vi "GetOpenLastSavedFileWhenStarting.vi"(5 "error in (no error)":errorcluster) -> (15 "OpenLastSavedFileWhenStarting":bool, 19 "error out":errorcluster)   [LabVIEW 2012, in "UmlEditor.lvclass"]
uses:
  <resource>/Framework/Providers/Open_GDS/UML/UmlEditor_class/UmlEditor.lvclass
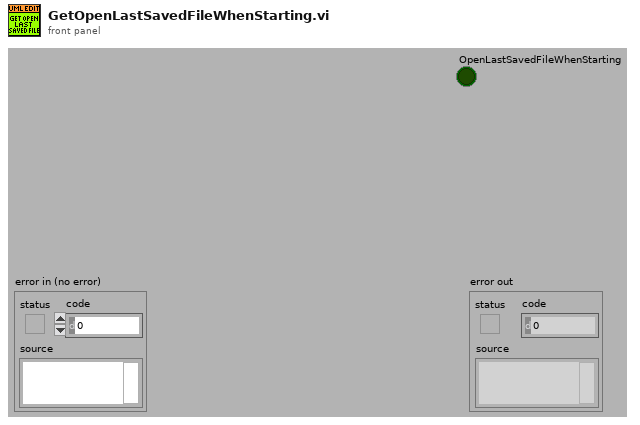
[diagram p1: front panel]
types:
  T1 = typedef "UmlEditor.lvclass/ObjectAttributes.ctl" = cluster{"ListeningQueueIn":refnum<queue>, "Event":refnum<user-event>, "UseProjectFolderAsBasePath":bool, "TypeSyncOption":bool, "Attr":string[], "ToolTip":cluster{"ToolTipOpen":bool, "LastToolTip":i32}, "ClassesToIgnore":string[], "UndoSize":i32, "OpenLastSavedFileWhenStarting":bool, "SyncOption":T2, "SyncTime(s)":i32, "Params":cluster{"IniParams":T3, "Value":string}[]}
  T2 = typedef "UMLEditor_SyncOptions.ctl" = cluster{"IgnoreInstrLib":bool, "IgnoreUserLib":bool, "IgnoreViLib":bool}
  T3 = typedef "UmlEditor.lvclass/IniParamsType.ctl" = enum16{"I have problem with UML stability on my computer"}
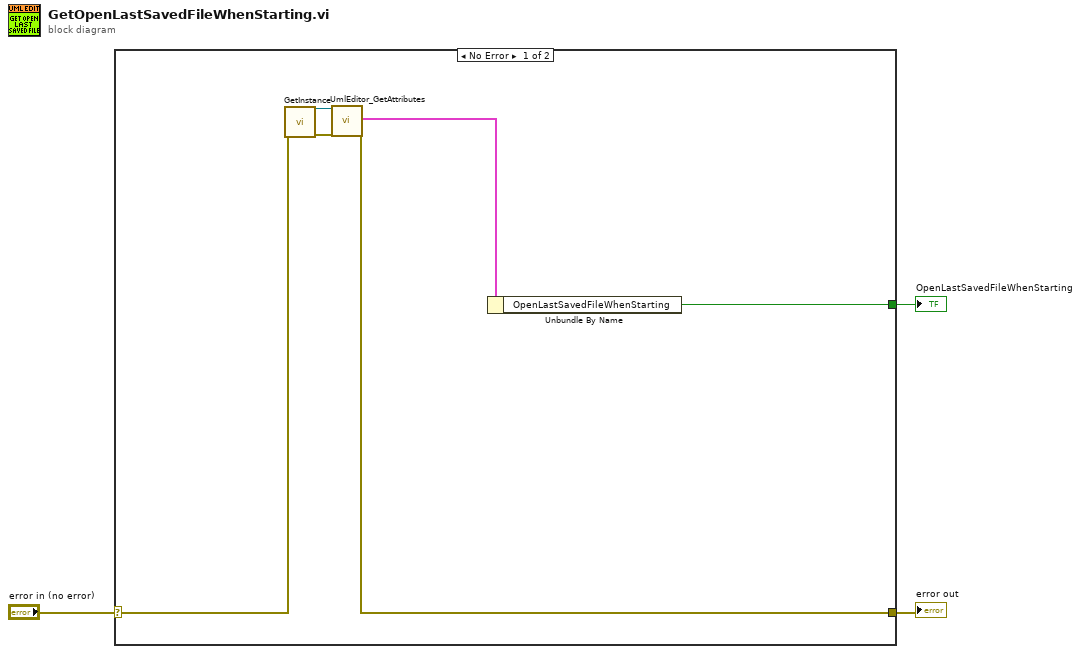
[diagram p0: block diagram]
diagram:
  n1 = case shown="No Error" "error in (no error)" {
    selector: "error in (no error)" -> [w5 w10]
    tunnel: [w8 w10] -> w2
    tunnel: [w7 _] -> w1
    frame No Error {
      n2 = call <resource>:"GetInstance.vi"("error in (no error)"=w5) -> ("reference out"=w6:refnum<class "UmlEditor.lvclass">, "error out"=w4:errorcluster)  [unwired: 17 out]
      n3 = call <resource>:"UmlEditor_GetAttributes.vi"("reference in"=w6, "error in (no error)"=w4) -> ("Attributes"=w9:T1, "error out"=w8:errorcluster)  [unwired: 14 in, 2 out]
      n4 = Unbundle By Name(w9) -> ("OpenLastSavedFileWhenStarting"=w7:bool)
    }
    frame Error {
    }
  }
  "error out" <- w2
  "OpenLastSavedFileWhenStarting" <- w1
